vi "getTriggering.vi"(8 "error in (no error)":errorcluster, 10 "triggering":string, 11 "K2602FileReader in":refnum<class "K2602FileReader.lvclass">) -> (0 "error out":errorcluster, 2 "triggering":T1(array[cluster]), 3 "K2602FileReader out":refnum<class "K2602FileReader.lvclass">)   [LabVIEW 2011, in "Tools.lvlib" / "Filing.lvlib" / "K2602FileReader.lvclass"]
uses:
  K2602FileReader.lvclass
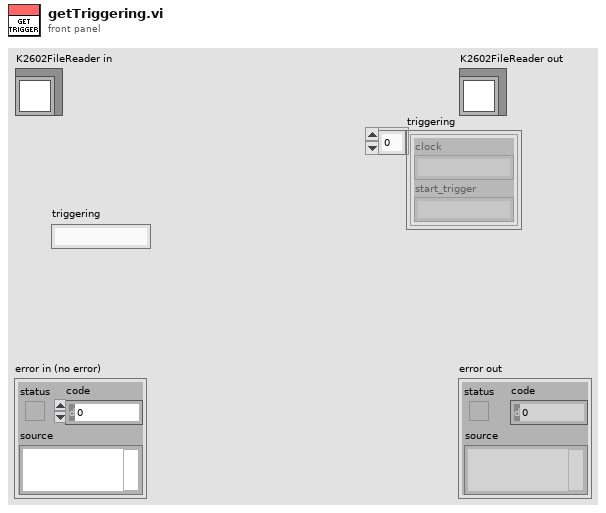
[diagram p1: front panel]
types:
  T1 = cluster{"clock":string, "start_trigger":string}[]
  T2 = cluster{"triggering":string, "triggering":string}
  T3 = cluster{"triggering":string, "triggering":string}[]
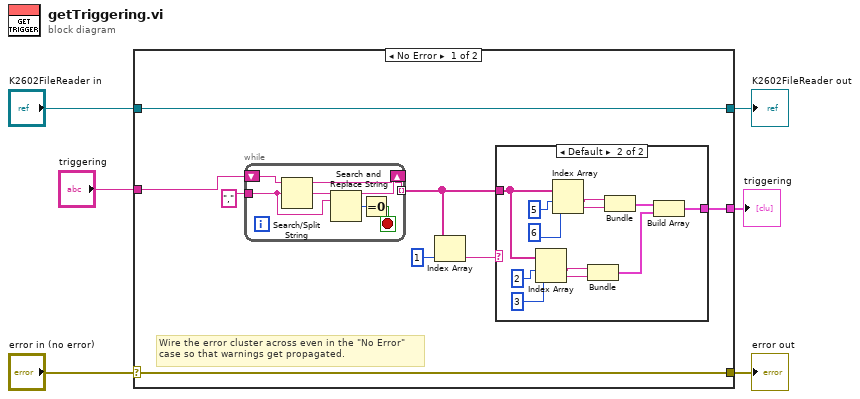
[diagram p0: block diagram]
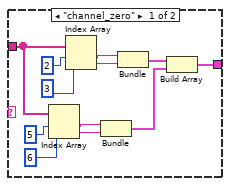
[diagram p2: hidden frame]
diagram:
  n1 = case shown="No Error" "error in (no error)" {
    selector: "error in (no error)" -> [w13 w47]
    tunnel: [w13 w47] -> w5
    tunnel: [w14 w46] -> w3
    tunnel: "K2602FileReader in" -> [w14 w46]
    tunnel: "triggering" -> [w11 _]
    tunnel: [w7 _] -> w1
    frame No Error {
      # "Wire the error cluster across even in the \"No Error\"\ncase so that warnings get propagated."
      n2 = while {
        tunnel: "," ("search string/char (-)") -> [w43]
        shift-right: [w41] -> _
        shift-left: w11 -> [w45]
        tunnel: [w39] -> w8 mode=indexing
        stop <- w42 stop-if-true
        n3 = Search/Split String(string=w45, search string/char (-)=w43) -> (substring before match=w39:string, match + rest of string=w44:string)  [unwired: 1 in, 1 out]
        n4 = Search and Replace String(input string=w44, search string=w43) -> (result string=w41:string, number of replacements=w40:i32)  [unwired: 6 in, 2 out]
        n5 = Equal To 0?(x=w40) -> (x = 0?=w42:bool)
      }
      n6 = Index Array(array=w8, index=1) -> (element=w9:string)
      n7 = case shown="Default" w9 {
        tunnel: w8 -> [w19 w31]
        tunnel: [w16 w28] -> w7
        frame "channel_zero" {
          n8 = Index Array(array=w19, index #1=5, index #2=6 ("index")) -> (element #1=w21:string, element #2=w20:string)
          n9 = Index Array(array=w19, index #1=2, index #2=3 ("index")) -> (element #1=w24:string, element #2=w23:string)
          n10 = Bundle("triggering"=w21, "triggering"=w20) -> (w17:T2)  [unwired: 1 in]
          n11 = Bundle("triggering"=w24, "triggering"=w23) -> (w18:T2)  [unwired: 1 in]
          n12 = Build Array(w18, w17) -> (w16:T3)
        }
        frame Default {
          n13 = Index Array(array=w31, index #1=2, index #2=3 ("index")) -> (element #1=w33:string, element #2=w32:string)
          n14 = Index Array(array=w31, index #1=5, index #2=6 ("index")) -> (element #1=w36:string, element #2=w35:string)
          n15 = Bundle("triggering"=w33, "triggering"=w32) -> (w29:T2)  [unwired: 1 in]
          n16 = Bundle("triggering"=w36, "triggering"=w35) -> (w30:T2)  [unwired: 1 in]
          n17 = Build Array(w30, w29) -> (w28:T3)
        }
      }
    }
    frame Error {
    }
  }
  "error out" <- w5
  "K2602FileReader out" <- w3
  "triggering" <- w1
